vi "ChangeInheritanceDialog.vi"(0 "ClassWriterGOOP300 in":refnum<class "ClassWriterNative.lvclass">, 1 "LvClass":refnum<vi>, 5 "error in (no error)":errorcluster) -> (14 "ClassWriterGOOP300 out":refnum<class "ClassWriterNative.lvclass">, 15 "BaseClassPath":path, 16 "Cancelled":bool, 19 "error out":errorcluster)   [LabVIEW 2012, in "ClassWriterNative.lvclass"]
uses:
  <resource>/Framework/Providers/Open_GDS/ClassProviders/Provider_LvNativeClass/ClassWriterNative_class/ClassWriterNative.lvclass
  <resource>/Framework/Providers/Open_GDS/SubVIs/GOOP_HelpButton.ctl
panel:
  in  "_HelpChangeInheritance":T1
  in  "_Cancel":bool
  in  "_OK":bool
  in  "_ChangeinheritanceToClass":u16(ring) caption="Change inheritance to this class"
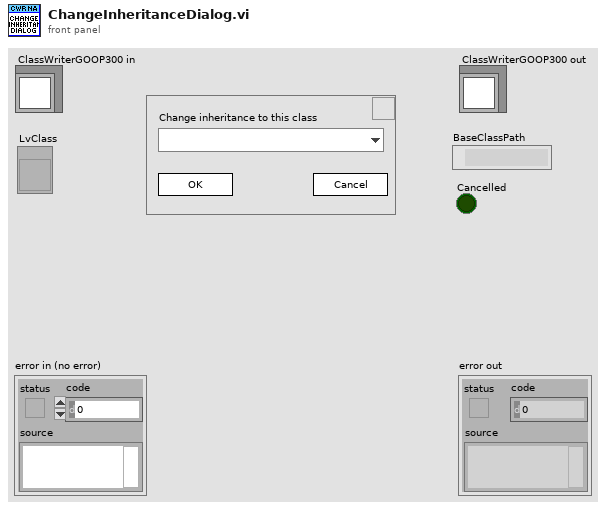
[diagram p1: front panel]
types:
  T1 = typedef "GOOP_HelpButton.ctl" = bool
  T2 = cluster{"LvClasses":refnum<vi>[], "ClassPathes":path[], "Cancelled":bool}
  T3 = typedef "GDSLvCLass_ClassSettingsType.ctl" = cluster{"ClassProviderName":string, "ClassTemplateUsed":string, "ClassTemplateVersion":string, "ClassDescription":string, "PlugIns":T4[], "ConnectorPanePattern":string}
  T4 = typedef "GDSLvClass_PlugIn.ctl" = cluster{"Type":T5, "ID":string, "Version":string, "Path":path, "Name":string, "Data":variant}
  T5 = typedef "GDSLvClass_PlugInTypes.ctl" = enum16{"DesignPattern", "MethodTypes"}
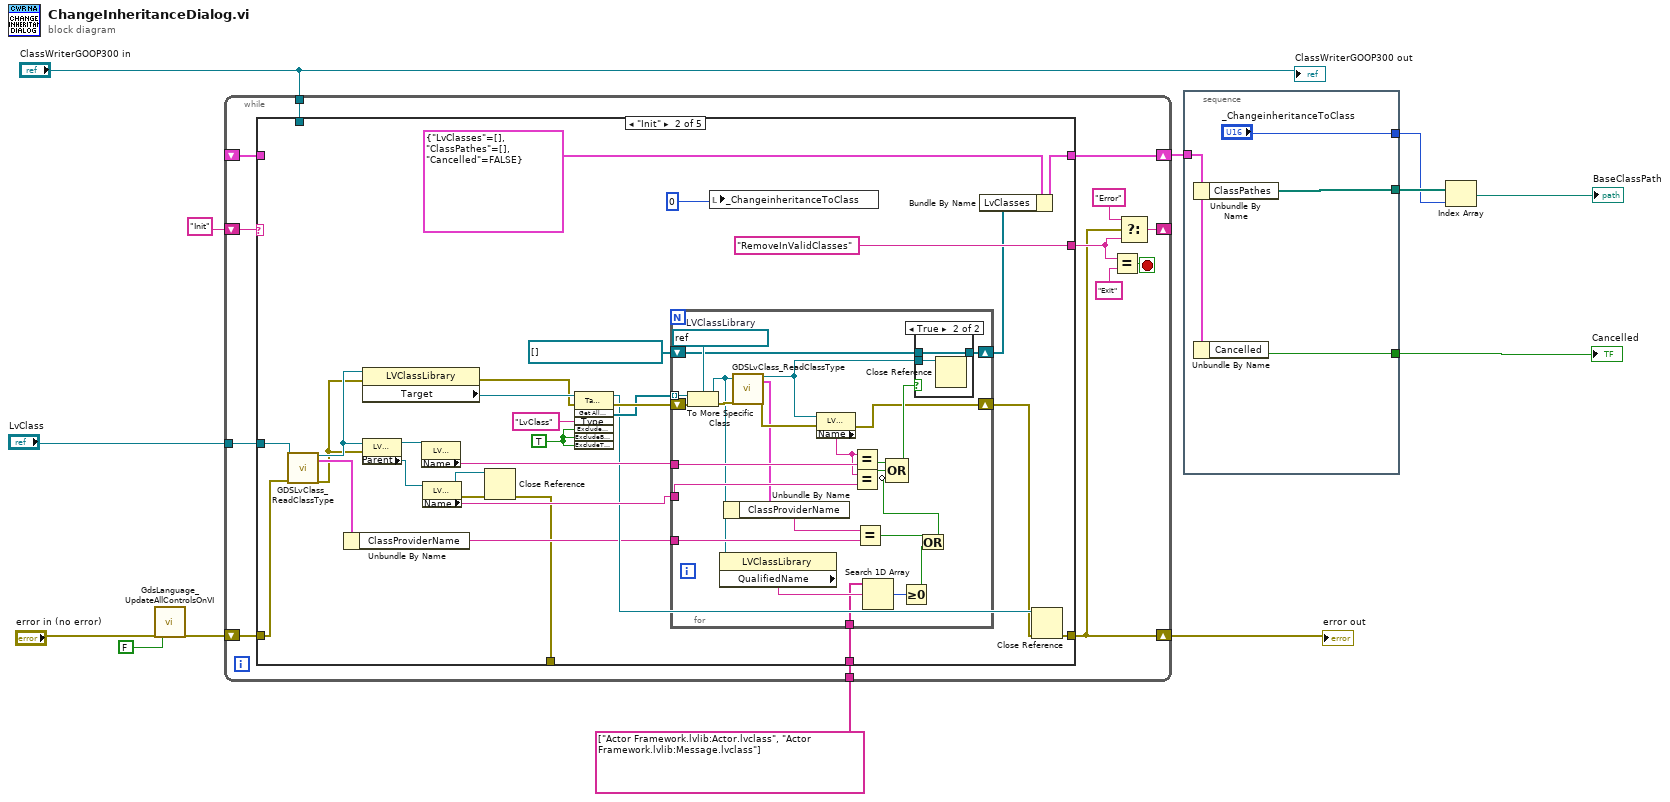
[diagram p0: block diagram]
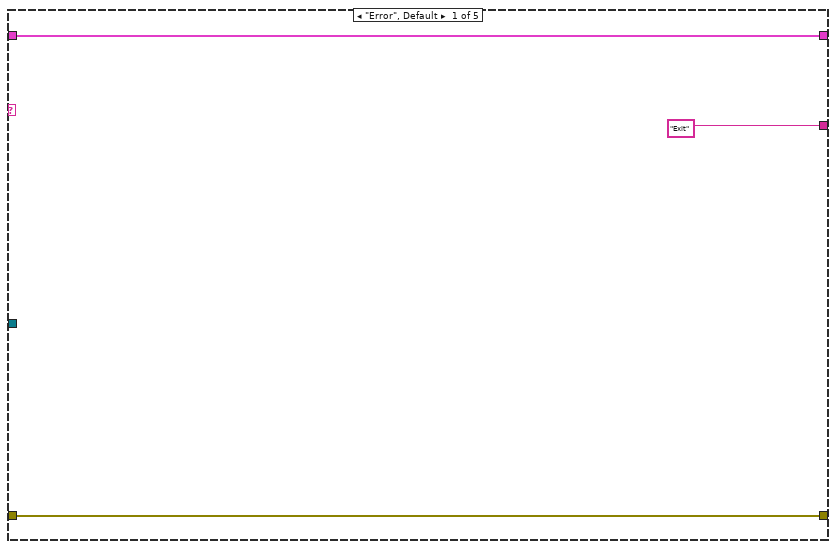
[diagram p2: hidden frame]
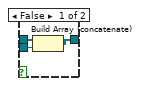
[diagram p3: hidden frame]
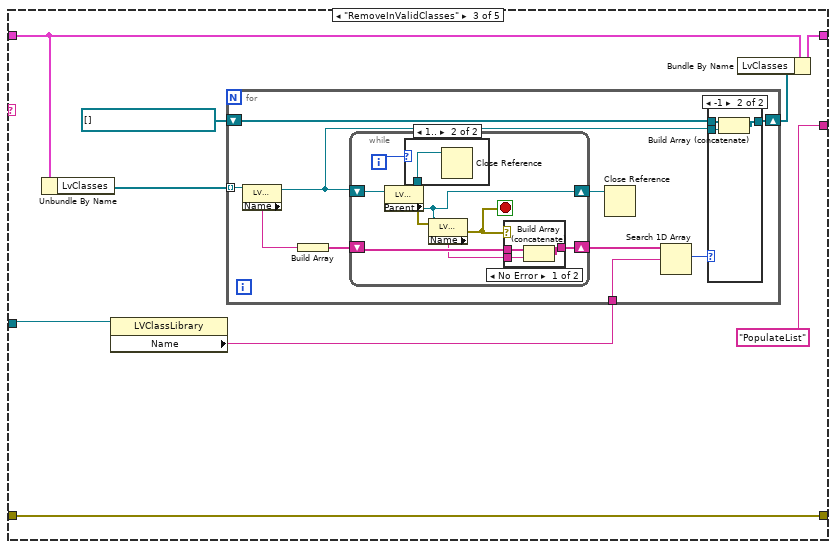
[diagram p4: hidden frame]
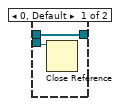
[diagram p5: hidden frame]
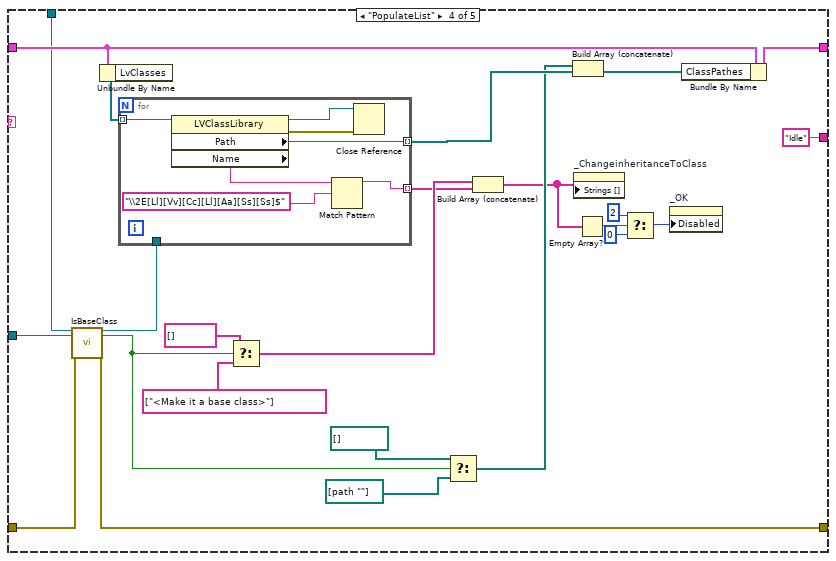
[diagram p8: hidden frame]
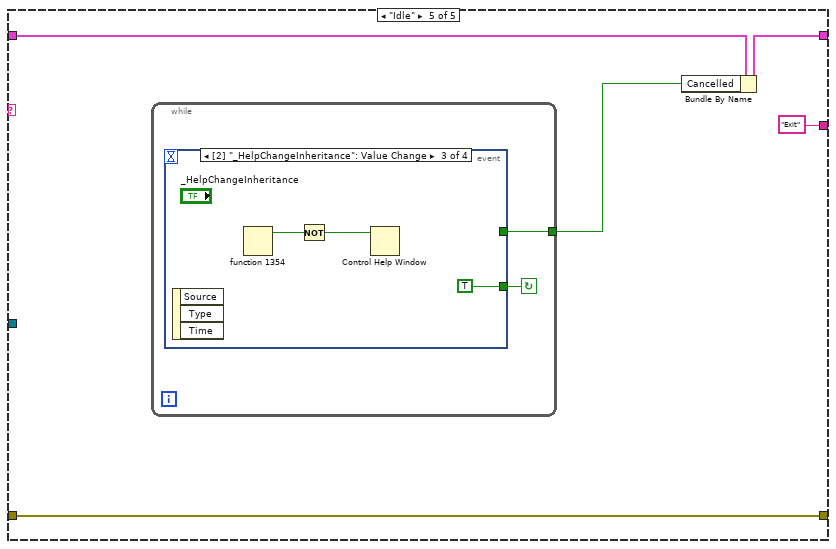
[diagram p9: hidden frame]
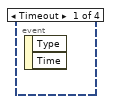
[diagram p10: hidden frame]
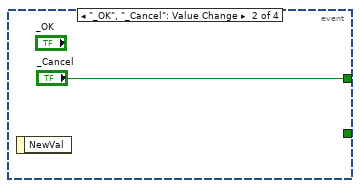
[diagram p11: hidden frame]
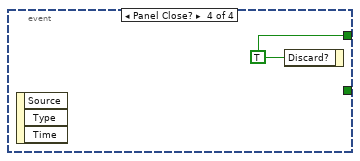
[diagram p12: hidden frame]
diagram:
  n1 = call <resource>:"GdsLanguage_UpdateAllControlsOnVI.vi"("error in (no error)"="error in (no error)", "CreateLanguageFile(Use this to create a languageFile)"=FALSE) -> ("error out"=w4:errorcluster)  [unwired: 16 in, 1 out]
  n2 = while {
    shift-right: [w19] -> w12
    shift-left: w4 -> [w26]
    shift-right: [w24] -> _
    shift-left: "Init" -> [w25]
    shift-right: [w18] -> w10
    shift-left: _ -> [w17]
    tunnel: "LvClass" -> [w16]
    tunnel: "ClassWriterGOOP300 in" -> [w15]
    tunnel: string[] ["Actor Framework.lvlib:Actor.lvclass", "Actor Framework.lvlib:Message.lvclass"] -> [w14]
    stop <- w23 stop-if-true
    n3 = case shown="\"Init\"" w25 {
      tunnel: w26 -> [w29 w39 w89 w129 w162]
      tunnel: [w29 w42 w89 w128 w162] -> w19
      tunnel: ["Exit" "RemoveInValidClasses" "PopulateList" "Idle" "Exit"] -> w20
      tunnel: [w27 w51 w91 w143 w160] -> w18
      tunnel: w17 -> [w27 _ w93 w144 w161]
      tunnel: w16 -> [_ w40 w96 w131 _]
      tunnel: w15 -> [_ _ _ w130 _]
      tunnel: [_ w34 _ _ _] -> _
      tunnel: w14 -> [_ w30 _ _ _]
      frame "Error", Default {
      }
      frame "Init" {
        w50 = TRUE ("ExcludeDependencies")
        n4 = call <resource>:"GDSLvClass_ReadClassType.vi"("Class Refnum In"=w40, "error in (no error)"=w39) -> ("Class Refnum Out"=w33:refnum<vi>, "ClassSettings"=w38:T3, "error out"=w32:errorcluster)  [unwired: 15 in]
        n5 = Unbundle By Name(w38) -> ("ClassProviderName"=w37:string)
        n6 = property class="LVClassLibrary"(reference=w33, error in=w32) -> (error out=w55:errorcluster, "Target"=w57:refnum<vi>)  [unwired: 1 out]
        n7 = property class="LVClassLibrary"(reference=w33, error in=w32) -> (reference out=w49:refnum<vi>, "Parent"=w48:refnum<vi>)  [unwired: 1 out]
        n8 = property class="LVClassLibrary"(reference=w49) -> ("Name"=w47:string)  [unwired: 1 in, 2 out]
        n9 = property class="LVClassLibrary"(reference=w48) -> (reference out=w35:refnum<vi>, error out=w36:errorcluster, "Name"=w46:string)  [unwired: 1 in]
        n10 = Close Reference(reference=w35, error in (no error)=w36) -> (error out=w34:errorcluster)
        n11 = invoke class="TargetItem" method="Get All Descendents"(reference=w57, error in=w55, "Type"="LvClass", "Exclude Dependencies"=w50, "ExcludeBuilds"=w50, "ExcludeTargets"=w50) -> (reference out=w41:refnum<vi>, error out=w54:errorcluster, "All Descendents"=w53:refnum<vi>[])  [unwired: 1 in, 4 out]
        n12 = for {
          shift-right: [w67] -> w31
          shift-left: w54 -> [w83]
          tunnel: w53 -> [w82] mode=indexing
          shift-right: [w73] -> w45
          shift-left: refnum<vi>[] [] -> [w74]
          tunnel: w47 -> [w80]
          tunnel: w46 -> [w78]
          tunnel: w37 -> [w68]
          tunnel: w30 -> [w63]
          w81 = refnum<vi> refnum  # LVClassLibrary
          n13 = To More Specific Class(target class=w81, reference=w82, error in=w83) -> (specific class reference=w65:refnum<vi>, error out=w70:errorcluster)
          n14 = property class="LVClassLibrary"(reference=w65) -> ("QualifiedName"=w64:string)  [unwired: 1 in, 2 out]
          n15 = call <resource>:"GDSLvClass_ReadClassType.vi"("Class Refnum In"=w65, "error in (no error)"=w70) -> ("Class Refnum Out"=w71:refnum<vi>, "ClassSettings"=w66:T3, "error out"=w72:errorcluster)  [unwired: 15 in]
          n16 = Unbundle By Name(w66) -> ("ClassProviderName"=w69:string)
          n17 = property class="LVClassLibrary"(reference=w71, error in=w72) -> (error out=w67:errorcluster, "Name"=w79:string)  [unwired: 1 out]
          n18 = Equal?(x=w79, y=w80) -> (x = y?=w76:bool)
          n19 = Equal?(x=w79, y=w78) -> (x = y?=w77:bool)
          n20 = Equal?(x=w69, y=w68) -> (x = y?=w61:bool)
          n21 = Search 1D Array(1D array=w63, element=w64) -> (index of element=w62:i32)  [unwired: 1 in]
          n22 = Greater Or Equal To 0?(x=w62) -> (x >= 0?=w60:bool)
          n23 = Or(x=w61, y=w60) -> (x .or. y?=w59:bool)
          n24 = Compound Arithmetic op=OR(w76, w77, invert w59) -> (w75:bool)
          n25 = case shown="True" w75 {
            tunnel: w74 -> [w86 w88]
            tunnel: [w85 w88] -> w73
            tunnel: w71 -> [w84 w87]
            frame False {
              n26 = Build Array (concatenate)(w86, w84) -> (w85:refnum<vi>[])
            }
            frame True {
              n27 = Close Reference(reference=w87) -> ()  [unwired: 1 in, 1 out]
            }
          }
        }
        n28 = local write "_ChangeinheritanceToClass"(u16 0) -> ()
        n29 = Bundle By Name(cluster=T2 {"LvClasses"=[], "ClassPathes"=[], "Cancelled"=FALSE}, "LvClasses"=w45) -> (w51:T2)
        n30 = Close Reference(reference=w41, error in (no error)=w31) -> (error out=w42:errorcluster)
      }
      frame "RemoveInValidClasses" {
        n31 = Unbundle By Name(w93) -> ("LvClasses"=w97:refnum<vi>[])
        n32 = property class="LVClassLibrary"(reference=w96) -> ("Name"=w95:string)  [unwired: 1 in, 2 out]
        n33 = for {
          tunnel: w97 -> [w107] mode=indexing
          tunnel: w95 -> [w102]
          shift-right: [w98] -> w92
          shift-left: refnum<vi>[] [] -> [w100]
          n34 = property class="LVClassLibrary"(reference=w107) -> (reference out=w99:refnum<vi>, "Name"=w105:string)  [unwired: 1 in, 1 out]
          n35 = Build Array(w105) -> (w104:string[])
          n36 = while {
            shift-right: [w115] -> w106
            shift-left: w99 -> [w121]
            shift-right: [w116] -> w103
            shift-left: w104 -> [w118]
            i -> [w113]
            stop <- w119 stop-if-true
            n37 = property class="LVClassLibrary"(reference=w121) -> (reference out=w114:refnum<vi>, error out=w120:errorcluster, "Parent"=w115:refnum<vi>)  [unwired: 1 in]
            n38 = case shown="1.." w113 {
              tunnel: w114 -> [_ w122]
              frame Default {
              }
              frame 1.. {
                n39 = Close Reference(reference=w122) -> ()  [unwired: 1 in, 1 out]
              }
            }
            n40 = property class="LVClassLibrary"(reference=w115, error in=w120) -> (error out=w119:errorcluster, "Name"=w117:string)  [unwired: 1 out]
            n41 = case shown="No Error" w119 {
              tunnel: w118 -> [w125 w126]
              tunnel: w117 -> [w124 _]
              tunnel: [w123 w126] -> w116
              frame No Error {
                n42 = Build Array (concatenate)(w125, w124) -> (w123:string[])
              }
              frame Error {
              }
            }
          }
          n43 = Close Reference(reference=w106) -> ()  [unwired: 1 in, 1 out]
          n44 = Search 1D Array(1D array=w103, element=w102) -> (index of element=w101:i32)  [unwired: 1 in]
          n45 = case shown="-1" w101 {
            tunnel: w100 -> [w108 w112]
            tunnel: w99 -> [w109 w111]
            tunnel: [w108 w110] -> w98
            frame 0, Default {
              n46 = Close Reference(reference=w109) -> ()  [unwired: 1 in, 1 out]
            }
            frame -1 {
              n47 = Build Array (concatenate)(w112, w111) -> (w110:refnum<vi>[])
            }
          }
        }
        n48 = Bundle By Name(cluster=w93, "LvClasses"=w92) -> (w91:T2)
      }
      frame "PopulateList" {
        n49 = call-dynamic "IsBaseClass.vi"("RefIn"=w130, "LvClass"=w131, "error in"=w129) -> ("RefOut"=w127:refnum<class "ClassWriterNative.lvclass">, "BaseClass"=w132:bool, "error out"=w128:errorcluster)  [unwired: 14 in]
        n50 = Unbundle By Name(w144) -> ("LvClasses"=w147:refnum<vi>[])
        n51 = for {
          tunnel: w147 -> [w157] mode=indexing
          tunnel: [w151] -> w146 mode=indexing
          tunnel: [w156] -> w142 mode=indexing
          tunnel: w127 -> [_]
          n52 = property class="LVClassLibrary"(reference=w157) -> (reference out=w154:refnum<vi>, error out=w155:errorcluster, "Path"=w156:path, "Name"=w153:string)  [unwired: 1 in]
          n53 = Match Pattern(string=w153, regular expression="\\2E[Ll][Vv][Cc][Ll][Aa][Ss][Ss]$") -> (before substring=w151:string)  [unwired: 1 in, 3 out]
          n54 = Close Reference(reference=w154, error in (no error)=w155) -> ()  [unwired: 1 out]
        }
        n55 = Select(t=string[] [], s=w132, f=string[] ["<Make it a base class>"] ("Strings []")) -> (s? t:f=w148:string[])
        n56 = Select(t=path[] [] ("array"), s=w132, f=path[] [path ""] ("array")) -> (s? t:f=w140:path[])
        n57 = Build Array (concatenate)(w148, w146) -> (w137:string[])
        n58 = Build Array (concatenate)(w140, w142) -> (w141:path[])
        n59 = property on="_ChangeinheritanceToClass" class="Ring (strict)"("Strings []"=w137) -> ()  [unwired: 2 in, 2 out]
        n60 = Empty Array?(array=w137) -> (empty?=w136:bool)
        n61 = Select(t=u8 2 ("Disabled"), s=w136, f=u8 0) -> (s? t:f=w135:u8)
        n62 = property on="_OK" class="Bool"("Disabled"=w135) -> ()  [unwired: 2 in, 2 out]
        n63 = Bundle By Name(cluster=w144, "ClassPathes"=w141) -> (w143:T2)
      }
      frame "Idle" {
        n64 = while {
          tunnel: [w164] -> w158
          stop <- w163 continue-if-true
          n65 = event shown="[2] \"_HelpChangeInheritance\": Value Change" {
            selector: _ -> [_ _ _ _]
            dyn-events: _ -> [_ _ _ _]
            timeout: _ -> [_ _ _ _]
            tunnel: [_ "_Cancel" _ w169] -> w164
            tunnel: [_ _ TRUE _] -> w163
            event Timeout {
              n66 = event-data() -> ()  [unwired: 1 in, 2 out]
            }
            event "_OK", "_Cancel": Value Change {
              n67 = event-data() -> ()  [unwired: 1 in, 1 out]
            }
            event Value Change {
              n68 = event-data() -> ()  [unwired: 1 in, 3 out]
              n69 = fn#1354() -> (1:w167:bool)  [unwired: 1 out]
              n70 = Not(x=w167) -> (.not. x?=w166:bool)
              n71 = Control Help Window(1:w166) -> ()  [unwired: 1 in]
            }
            event Panel Close? {
              w169 = TRUE ("Discard?")
              n72 = event-data() -> ()  [unwired: 1 in, 3 out]
              n73 = event-data("Discard?"=w169) -> ()  [unwired: 1 in, 1 out]
            }
          }
        }
        n74 = Bundle By Name(cluster=w161, "Cancelled"=w158) -> (w160:T2)
      }
    }
    n75 = Equal?(x=w20, y="Exit") -> (x = y?=w23:bool)
    n76 = Select(t="Error", s=w19, f=w20) -> (s? t:f=w24:string)
  }
  "error out" <- w12
  n77 = stacked-sequence {
    tunnel: w10 -> [w171]
    tunnel: ["_ChangeinheritanceToClass"] -> w6
    tunnel: [w172] -> w9
    tunnel: [w170] -> w7
    frame #0 {
      n78 = Unbundle By Name(w171) -> ("ClassPathes"=w172:path[])
      n79 = Unbundle By Name(w171) -> ("Cancelled"=w170:bool)
    }
  }
  "Cancelled" <- w7
  n80 = Index Array(array=w9, index=w6) -> (element=→"BaseClassPath":path)
  "ClassWriterGOOP300 out" <- "ClassWriterGOOP300 in"
